vi "set_acceleration.vi"(8 "error in (no error)":errorcluster, 10 "Acceleration (step/sec^2)":i32, 11 "Newport Model 8742 in":refnum<class "Newport Model 8742.lvclass">) -> (0 "error out":errorcluster, 3 "Newport Model 8742 out":refnum<class "Newport Model 8742.lvclass">)   [LabVIEW 2020, in "Newport Model 8742.lvclass"]
uses:
  Newport Model 8742.lvclass
  Newport Model 8742.lvclass/Newport Model 8742.ctl
  Picomotor/Picomotor.lvclass
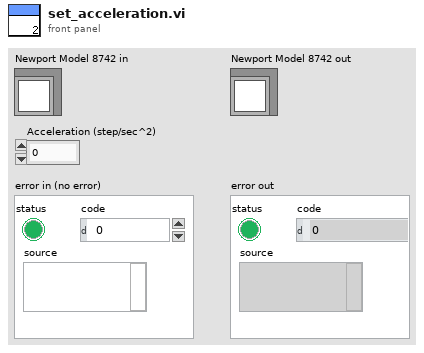
[diagram p1: front panel]
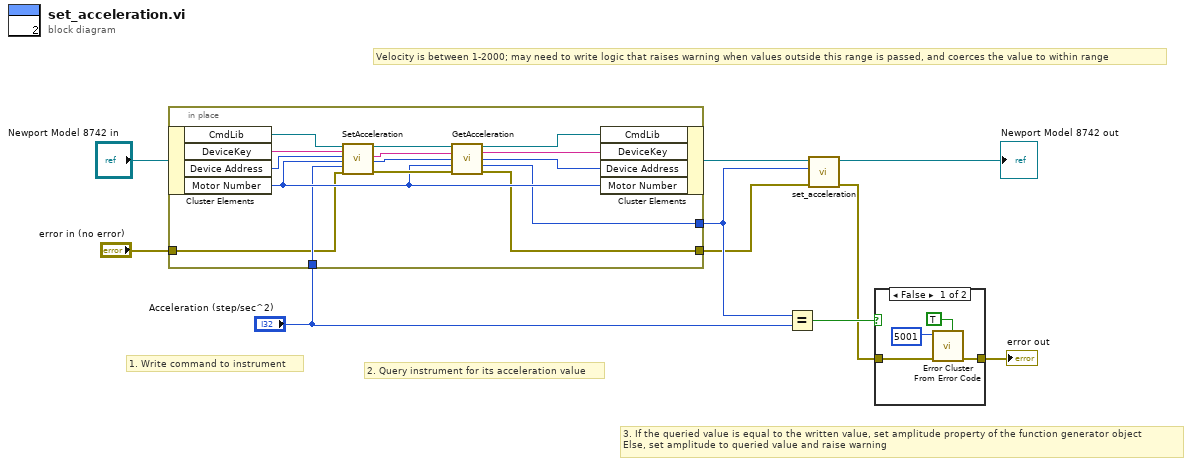
[diagram p0: block diagram]
diagram:
  # "Velocity is between 1-2000; may need to write logic that raises warning when values outside this range is passed, and coerces the value to within range"
  # "3. If the queried value is equal to the written value, set amplitude property of the function generator object\nElse, set amplitude to queried value and raise warning"
  # "2. Query instrument for its acceleration value"
  # "1. Write command to instrument"
  n1 = in-place {
    in-place-border: "error in (no error)" -> [w13]
    in-place-border: "Acceleration (step/sec^2)" -> [w14]
    in-place-border: [w12] -> w4
    in-place-border: [w11] -> w3
    n2 = in-place-cluster #1("Newport Model 8742 in") -> ("CmdLib"=w25:refnum<k24>, "DeviceKey"=w24:string, "Device Address"=w23:i32, "Motor Number"=w15:i32)
    n3 = call <instrlib>:"SetAcceleration.vi"("CmdLib In"=w25, "DeviceKey In"=w24, "Device Address In"=w23, "Motor"=w15, "Steps Per Sec 2"=w14, "error in (no error)"=w13) -> ("CmdLib Out"=w22:refnum<k24>, "DeviceKey Out"=w21:string, "Device Address Out"=w20:i32, "error out"=w19:errorcluster)  [unwired: 10 in]
    n4 = call <instrlib>:"GetAcceleration.vi"("CmdLib In"=w22, "DeviceKey In"=w21, "Device Address In"=w20, "Motor"=w15, "error in (no error)"=w19) -> ("CmdLib Out"=w18:refnum<k24>, "DeviceKey Out"=w17:string, "Device Address Out"=w16:i32, "Steps Per Sec 2"=w12:i32, "error out"=w11:errorcluster)  [unwired: 6 in]
    n5 = in-place-cluster #1("CmdLib"=w18, "DeviceKey"=w17, "Device Address"=w16, "Motor Number"=w15) -> (w7:refnum<class "Newport Model 8742.lvclass">)
  }
  n6 = Equal?(x=w4, y="Acceleration (step/sec^2)") -> (x = y?=w5:bool)
  n7 = call-parent "set_acceleration.vi"("error in (no error)"=w3, "Acceleration (steps/sec^2)"=w4, "Picomotor in"=w7) -> ("error out"=w2:errorcluster, "Picomotor out"=→"Newport Model 8742 out":refnum<class "Newport Model 8742.lvclass">)  [unwired: 7 in]
  n8 = case shown="False" w5 {
    tunnel: [w28 w30] -> w1
    tunnel: w2 -> [w26 w30]
    frame False {
      n9 = call <vilib>:"Error Cluster From Error Code.vi"("is warning? (False)"=TRUE, "error in (no error)"=w26, "error code (0)"=5001) -> ("error out"=w28:errorcluster)  [unwired: 6 in]
    }
    frame True {
    }
  }
  "error out" <- w1
